vi "Iso Measurement Write.vi"(8 "error in":errorcluster, 10 "Iso Measurement STS":i32, 11 "Cycler in":refnum<class "Cycler.lvclass">) -> (0 "error out":errorcluster, 3 "Cycler out":refnum<class "Cycler.lvclass">)   [LabVIEW 2023, in "Cycler.lvclass"]
uses:
  Cycler.lvclass
  Cycler.lvclass/Cycler.ctl
  Low Level Capabilities/Iso Measurement/Iso Measurement.lvclass
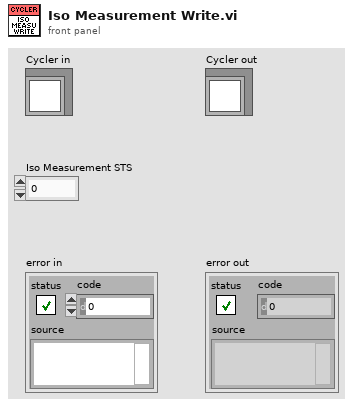
[diagram p1: front panel]
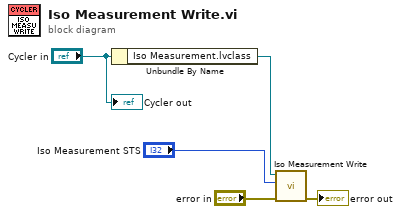
[diagram p0: block diagram]
diagram:
  n1 = Unbundle By Name("Cycler in") -> ("Iso Measurement.lvclass"=w1:refnum<class "Iso Measurement.lvclass">)
  n2 = call-dynamic "Iso Measurement Write.vi"("error in"="error in", "Iso Measurement STS"="Iso Measurement STS", "Iso Measurement in"=w1) -> ("error out"=→"error out":errorcluster)  [unwired: 7 in, 1 out]
  "Cycler out" <- "Cycler in"
